vi "Array Investigation Part 4.vi"() -> ()   [LabVIEW 2010]
doc: "This VI is an exercise in the LabVIEW Core I course.\n\nEnter the number of columns and rows you want generated, then run the VI. This VI generates an array with the number of rows and columns you specify."
panel:
  out "Second Column":dbl[](array[numeric])
  out "Third Row":dbl[](array[numeric])
  out "Array":dbl[][](array[numeric])
  in  "Rows":i32=80
  in  "Columns":i32=80
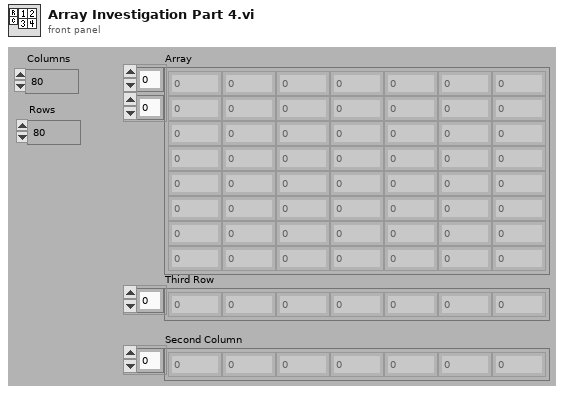
[diagram p1: front panel]
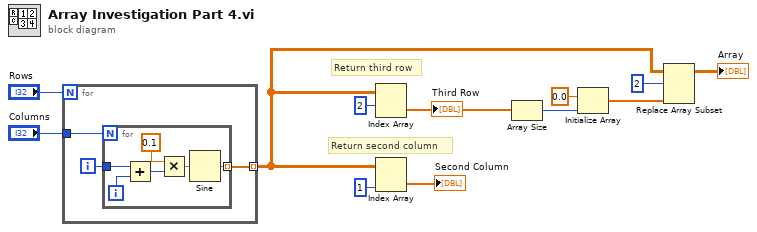
[diagram p0: block diagram]
diagram:
  # "Return second column"
  # "Return third row"
  n1 = for {
    N: "Rows" -> [_]
    tunnel: [w15] -> w5 mode=indexing
    tunnel: "Columns" -> [w14]
    i -> [w13]
    n2 = for {
      N: w14 -> [_]
      tunnel: [w21] -> w15 mode=indexing
      tunnel: w13 -> [w18]
      i -> [w19]
      n3 = Add(x=w18, y=w19) -> (x+y=w20:i32)
      n4 = Multiply(x=0.1, y=w20) -> (x*y=w17:dbl)
      n5 = Sine(x=w17) -> (sin(x)=w21:dbl)
    }
  }
  n6 = Index Array(array=w5, index (row)=2) -> (element=w2:dbl[])  [unwired: 1 in]
  "Third Row" <- w2
  n7 = Index Array(array=w5, index (col)=1 ("disabled index (col)")) -> (element=→"Second Column":dbl[])  [unwired: 1 in]
  n8 = Array Size(array=w2) -> (size(s)=w8:i32)
  n9 = Initialize Array(0.0 ("element"), w8) -> (w6:dbl[])
  n10 = Replace Array Subset(array=w5, new element=w6, index (row)=2 ("disabled index (col)")) -> (→"Array":dbl[][])  [unwired: 1 in]
